vi "GET_AllKeys.vi"() -> ()   [LabVIEW 2020]
uses:
  <vilib>/Utility/config.llb/NI_LVConfig.lvlib
  <vilib>/Utility/config.llb/Read Key (Boolean).vi
  <vilib>/Utility/config.llb/Read Key (Double).vi
  <vilib>/Utility/config.llb/Read Key (I32).vi
  <vilib>/Utility/config.llb/Read Key (Path).vi
  <vilib>/Utility/config.llb/Read Key (String).vi
  <vilib>/Utility/config.llb/Read Key (U32).vi
panel:
  out "error out":errorcluster
  in  "error in (no error)":errorcluster
  in  "Configuration file path":path
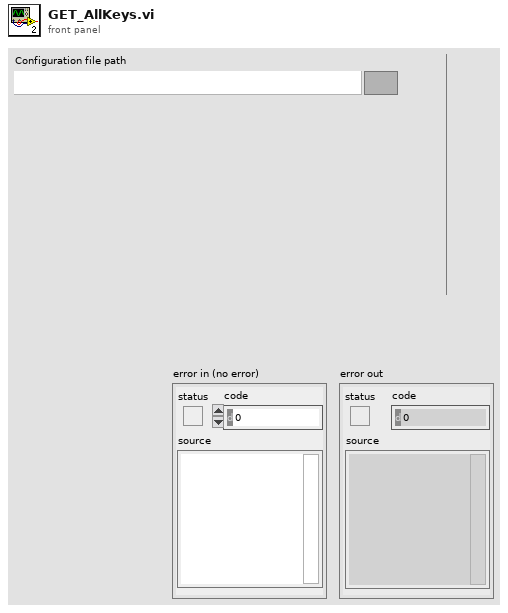
[diagram p1: front panel]
types:
  T1 = typedef "NI_LVConfig.lvlib/Config Data RefNum.ctl" = refnum<k1>
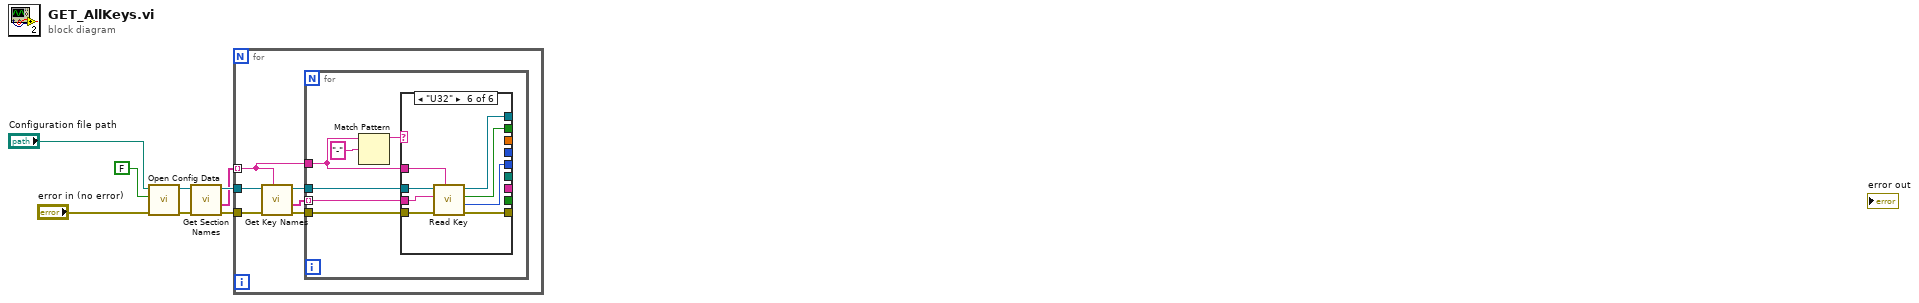
[diagram p0: block diagram]
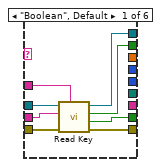
[diagram p2: hidden frame]
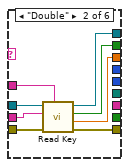
[diagram p3: hidden frame]
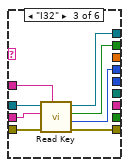
[diagram p4: hidden frame]
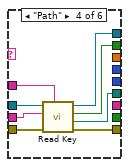
[diagram p5: hidden frame]
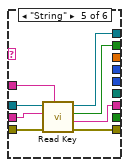
[diagram p6: hidden frame]
diagram:
  n1 = call <vilib>:"Open Config Data.vi"("error in (no error)"="error in (no error)", "create file if necessary (T)"=FALSE, "configuration file path"="Configuration file path") -> ("error out"=w4:errorcluster, "refnum"=w5:T1)  [unwired: 6 in, 1 out]
  n2 = call <vilib>:"Get Section Names.vi"("error in (no error)"=w4, "refnum"=w5) -> ("error out"=w1:errorcluster, "section names"=w2:string[], "refnum out"=w3:T1)  [unwired: 7 in]
  n3 = for {
    tunnel: w3 -> [w14]
    tunnel: w2 -> [w10] mode=indexing
    tunnel: w1 -> [w13]
    n4 = call <vilib>:"Get Key Names.vi"("section"=w10, "error in (no error)"=w13, "refnum"=w14) -> ("error out"=w9:errorcluster, "key names"=w12:string[], "refnum out"=w11:T1)  [unwired: 5 in, 1 out]
    n5 = for {
      tunnel: w12 -> [w17] mode=indexing
      tunnel: w11 -> [w18]
      tunnel: w10 -> [w16]
      tunnel: w9 -> [w15]
      n6 = Match Pattern(string=w16, regular expression="-") -> (before substring=w19:string)  [unwired: 1 in, 3 out]
      n7 = case shown="\"U32\"" w19 {
        tunnel: w18 -> [w28 w35 w43 w50 w58 w64]
        tunnel: w17 -> [w27 w36 w44 w52 w60 w66]
        tunnel: w16 -> [w26 w34 w42 w51 w59 w65]
        tunnel: w15 -> [w25 w33 w38 w45 w57 w68]
        tunnel: [w24 w32 w37 w46 w55 w67] -> _
        tunnel: [w23 w31 w41 w49 w54 w62] -> _
        tunnel: [_ w30 _ _ _ _] -> _
        tunnel: [w22 w29 w40 w47 w53 w61] -> _
        tunnel: [_ _ w39 _ _ _] -> _
        tunnel: [w21 _ _ _ _ _] -> _
        tunnel: [_ _ _ w48 _ _] -> _
        tunnel: [_ _ _ _ w56 _] -> _
        tunnel: [_ _ _ _ _ w63] -> _
        frame "Boolean", Default {
          n8 = call-poly <vilib>:"Read Key.vi"("section"=w26, "error in (no error)"=w25, "key"=w27, "refnum"=w28) -> ("error out"=w24:errorcluster, "value"=w21:bool, "found?"=w22:bool, "refnum out"=w23:T1)  [unwired: 4 in]
        }
        frame "Double" {
          n9 = call-poly <vilib>:"Read Key.vi"("section"=w34, "error in (no error)"=w33, "key"=w36, "refnum"=w35) -> ("error out"=w32:errorcluster, "value"=w30:dbl, "found?"=w29:bool, "refnum out"=w31:T1)  [unwired: 4 in]
        }
        frame "I32" {
          n10 = call-poly <vilib>:"Read Key.vi"("section"=w42, "error in (no error)"=w38, "key"=w44, "refnum"=w43) -> ("error out"=w37:errorcluster, "value"=w39:i32, "found?"=w40:bool, "refnum out"=w41:T1)  [unwired: 4 in]
        }
        frame "Path" {
          n11 = call-poly <vilib>:"Read Key.vi"("section"=w51, "error in (no error)"=w45, "key"=w52, "refnum"=w50) -> ("error out"=w46:errorcluster, "value"=w48:path, "found?"=w47:bool, "refnum out"=w49:T1)  [unwired: 4 in]
        }
        frame "String" {
          n12 = call-poly <vilib>:"Read Key.vi"("section"=w59, "error in (no error)"=w57, "key"=w60, "refnum"=w58) -> ("error out"=w55:errorcluster, "value"=w56:string, "found?"=w53:bool, "refnum out"=w54:T1)  [unwired: 4 in]
        }
        frame "U32" {
          n13 = call-poly <vilib>:"Read Key.vi"("section"=w65, "error in (no error)"=w68, "key"=w66, "refnum"=w64) -> ("error out"=w67:errorcluster, "value"=w63:u32, "found?"=w61:bool, "refnum out"=w62:T1)  [unwired: 4 in]
        }
      }
    }
  }
